vi "Close All Ref.vi"(8 "error in (no error)":errorcluster, 11 "Control references":T1(array[cluster])) -> (0 "error out":errorcluster)   [LabVIEW 2019]
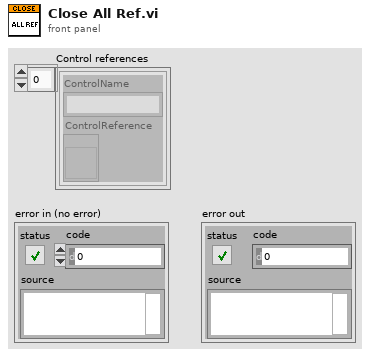
[diagram p1: front panel]
types:
  T1 = cluster{"ControlName":string, "ControlReference":refnum<vi>}[]
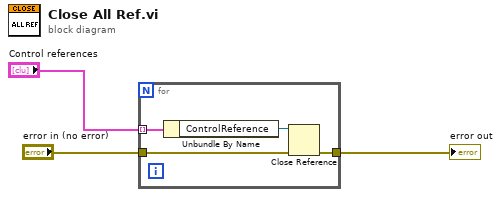
[diagram p0: block diagram]
diagram:
  n1 = for {
    tunnel: "Control references" -> [w7] mode=indexing
    tunnel: "error in (no error)" -> [w5]
    tunnel: [w4] -> w3
    n2 = Unbundle By Name(w7) -> ("ControlReference"=w6:refnum<vi>)
    n3 = Close Reference(reference=w6, error in (no error)=w5) -> (error out=w4:errorcluster)
  }
  "error out" <- w3
